vi "tag bus to profibus.vi"(10 "slave configuration":T2, 11 "data table in in":T1) -> (1 "Data":u8[](array[numeric]), 2 "slave index":i8, 3 "data table out":T1)   [LabVIEW 2013, in "Profibus Module runtime.lvclass"]
uses:
  Profibus Module runtime.lvclass
  profibus slave configuration.ctl
  profibus mapping configuration.ctl
  <vilib>/NI/Tag Bus/tag/Data Type.ctl
  <vilib>/NI/Tag Bus/table/data table.ctl
  <vilib>/NI/Tag Bus/table/data polymorphs/read one/read Double.vi
  <vilib>/NI/Tag Bus/table/data polymorphs/read one/read Single.vi
  <vilib>/NI/Tag Bus/table/data polymorphs/read one/read U32.vi
  <vilib>/NI/Tag Bus/table/data polymorphs/read one/read U16.vi
  <vilib>/NI/Tag Bus/table/data polymorphs/read one/read I16.vi
  <vilib>/NI/Tag Bus/table/data polymorphs/read one/read Array of U8.vi
  <vilib>/NI/Tag Bus/table/data polymorphs/read one/read Array of U32.vi
  <vilib>/NI/Tag Bus/table/data polymorphs/read one/read Array of U16.vi
  <vilib>/NI/Tag Bus/table/data polymorphs/read one/read U8.vi
  <vilib>/NI/Tag Bus/table/data polymorphs/read one/read I8.vi
  <vilib>/NI/Tag Bus/table/data polymorphs/read one/read Boolean.vi
  <vilib>/NI/Tag Bus/table/data table.lvlib
  <vilib>/NI/Tag Bus/tag/tag descriptor.lvclass
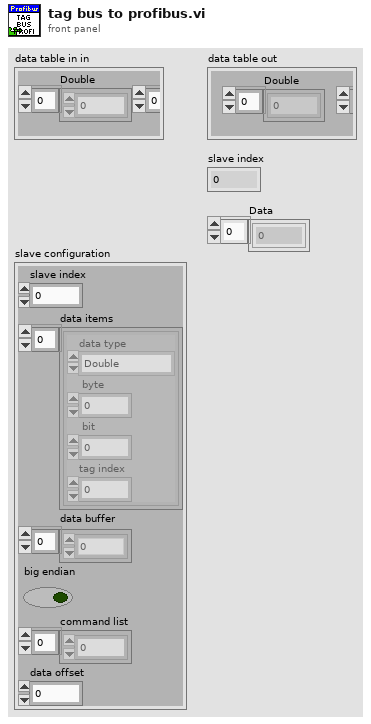
[diagram p1: front panel]
types:
  T1 = typedef "tag bus.lvlib/data table.lvlib/data table.ctl" = cluster{"Double":dbl[], "Single":sgl[], "I64":i64[], "I32":i32[], "I16":i16[], "I8":i8[], "U64":u64[], "U32":u32[], "U16":u16[], "U8":u8[], "Boolean":bool[], "String":string[], "Array of Double":cluster{"DBL Array":dbl[]}[], "Array of Single":cluster{"SGL Array":sgl[]}[], "Array of I64":cluster{"I64 Array":i64[]}[], "Array of I32":cluster{"I32 Array":i32[]}[], "Array of I16":cluster{"I16 Array":i16[]}[], "Array of I8":cluster{"I8 Array":i8[]}[], "Array of U64":cluster{"U64 Array":u64[]}[], "Array of U32":cluster{"U32 Array":u32[]}[], "Array of U16":cluster{"U16 Array":u16[]}[], "Array of U8":cluster{"U8 Array":u8[]}[], "Array of Boolean":cluster{"Boolean Array":bool[]}[], "Array of String":cluster{"String Array":string[]}[]}
  T2 = typedef "Profibus Module runtime.lvclass/profibus slave configuration.ctl" = cluster{"slave index":i8, "data items":T3[], "data buffer":u8[], "big endian":bool, "command list":u32[], "data offset":u8}
  T3 = typedef "Profibus Module runtime.lvclass/profibus mapping configuration.ctl" = cluster{"data type":T4, " byte":i32, " bit":i32, "tag index":i32}
  T4 = typedef "tag bus.lvlib/tag descriptor.lvclass/Data Type.ctl" = enum16{"Double", "Single", "I64", "I32", "I16", "I8", "U64", "U32", "U16", "U8", "Boolean", "String", "Array of Double", "Array of Single", "Array of I64", "Array of I32", "Array of I16", "Array of I8", "Array of U64", "Array of U32", "Array of U16", "Array of U8", "Array of Boolean", "Array of String"}
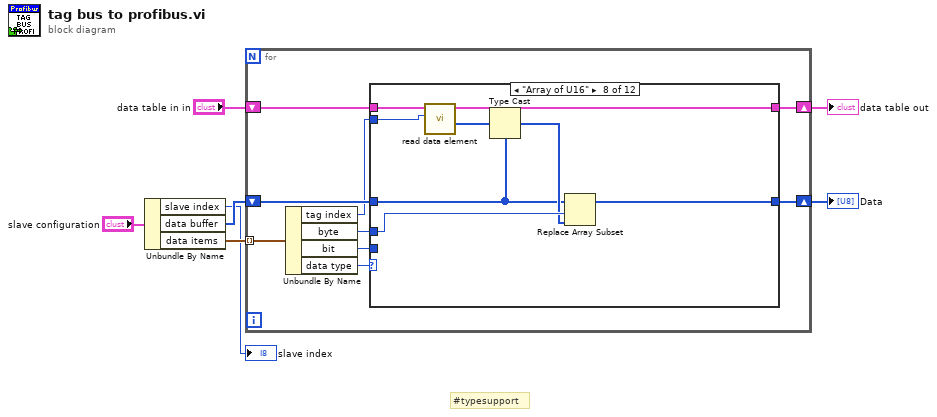
[diagram p0: block diagram]
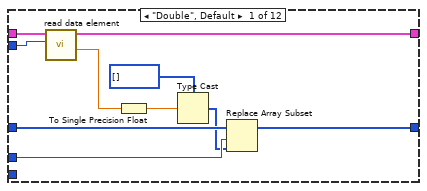
[diagram p2: hidden frame]
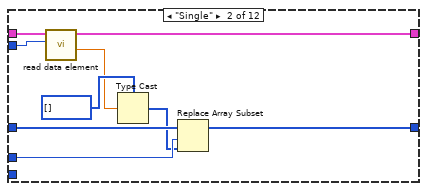
[diagram p3: hidden frame]
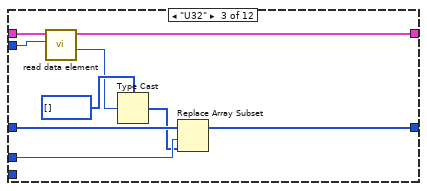
[diagram p4: hidden frame]
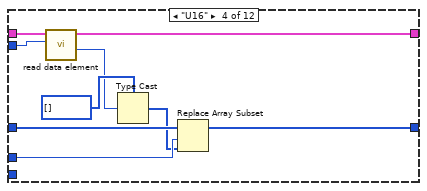
[diagram p5: hidden frame]
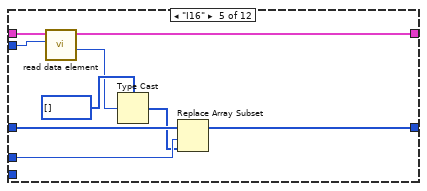
[diagram p6: hidden frame]
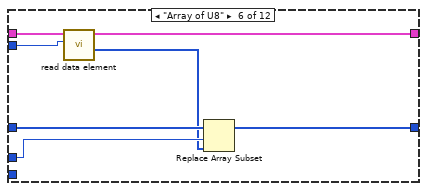
[diagram p7: hidden frame]
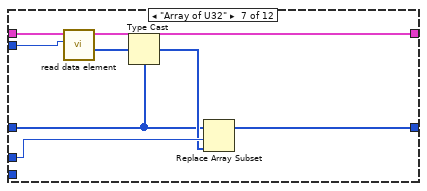
[diagram p8: hidden frame]
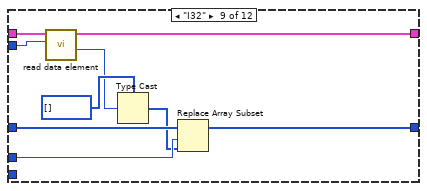
[diagram p9: hidden frame]
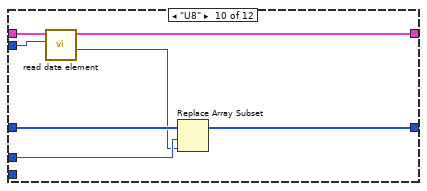
[diagram p10: hidden frame]
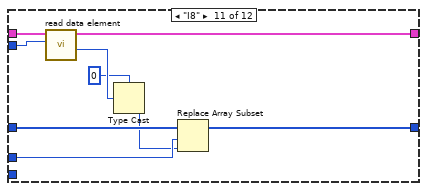
[diagram p11: hidden frame]
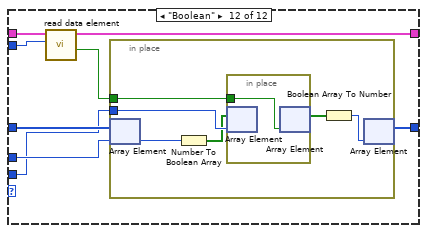
[diagram p12: hidden frame]
diagram:
  # "#typesupport"
  n1 = Unbundle By Name("slave configuration") -> ("slave index"=→"slave index":i8, "data buffer"=w6:u8[], "data items"=w4:T3[])
  n2 = for {
    tunnel: w4 -> [w16] mode=indexing
    shift-right: [w14] -> w5
    shift-left: w6 -> [w15]
    shift-right: [w9] -> w2
    shift-left: "data table in in" -> [w10]
    n3 = Unbundle By Name(w16) -> ("tag index"=w8:i32, "byte"=w13:i32, "bit"=w11:i32, "data type"=w12:T4)
    n4 = case shown="\"Array of U16\"" w12 {
      tunnel: w8 -> [w18 w28 w37 w46 w55 w68 w76 w84 w87 w96 w105 w111]
      tunnel: w15 -> [w24 w34 w43 w52 w61 w66 w70 w78 w93 w101 w110 w118]
      tunnel: w13 -> [w22 w32 w41 w50 w59 w64 w73 w81 w91 w99 w108 w117]
      tunnel: [w23 w33 w42 w51 w60 w65 w74 w82 w92 w100 w109 w116] -> w14
      tunnel: w11 -> [_ _ _ _ _ _ _ _ _ _ _ w115]
      tunnel: w10 -> [w20 w30 w39 w48 w57 w69 w77 w85 w89 w98 w107 w112]
      tunnel: [w19 w29 w38 w47 w56 w67 w75 w83 w88 w97 w106 w113] -> w9
      frame "Double", Default {
        n5 = call-poly <vilib>:"read data element.vi"("index"=w18, "data table in"=w20) -> ("value"=w17:dbl, "data table out"=w19:T1)  [unwired: 8 in]
        n6 = To Single Precision Float(number=w17) -> (single precision float=w25:sgl)
        n7 = Type Cast(type=u8[] [] ("Array 2"), x=w25) -> (*(type *) &x=w21:u8[])
        n8 = Replace Array Subset(array=w24, new element=w21, index=w22) -> (w23:u8[])
      }
      frame "Single" {
        n9 = call-poly <vilib>:"read data element.vi"("index"=w28, "data table in"=w30) -> ("value"=w27:sgl, "data table out"=w29:T1)  [unwired: 8 in]
        n10 = Type Cast(type=u8[] [] ("Array 2"), x=w27) -> (*(type *) &x=w31:u8[])
        n11 = Replace Array Subset(array=w34, new element=w31, index=w32) -> (w33:u8[])
      }
      frame "U32" {
        n12 = call-poly <vilib>:"read data element.vi"("index"=w37, "data table in"=w39) -> ("value"=w36:u32, "data table out"=w38:T1)  [unwired: 8 in]
        n13 = Type Cast(type=u8[] [] ("Array 2"), x=w36) -> (*(type *) &x=w40:u8[])
        n14 = Replace Array Subset(array=w43, new element=w40, index=w41) -> (w42:u8[])
      }
      frame "U16" {
        n15 = call-poly <vilib>:"read data element.vi"("index"=w46, "data table in"=w48) -> ("value"=w45:u16, "data table out"=w47:T1)  [unwired: 8 in]
        n16 = Type Cast(type=u8[] [] ("Array 2"), x=w45) -> (*(type *) &x=w49:u8[])
        n17 = Replace Array Subset(array=w52, new element=w49, index=w50) -> (w51:u8[])
      }
      frame "I16" {
        n18 = call-poly <vilib>:"read data element.vi"("index"=w55, "data table in"=w57) -> ("value"=w54:i16, "data table out"=w56:T1)  [unwired: 8 in]
        n19 = Type Cast(type=u8[] [] ("Array 2"), x=w54) -> (*(type *) &x=w58:u8[])
        n20 = Replace Array Subset(array=w61, new element=w58, index=w59) -> (w60:u8[])
      }
      frame "Array of U8" {
        n21 = call-poly <vilib>:"read data element.vi"("index"=w68, "data table in"=w69) -> ("value"=w63:u8[], "data table out"=w67:T1)  [unwired: 8 in]
        n22 = Replace Array Subset(array=w66, new element=w63, index=w64) -> (w65:u8[])
      }
      frame "Array of U32" {
        n23 = call-poly <vilib>:"read data element.vi"("index"=w76, "data table in"=w77) -> ("value"=w72:u32[], "data table out"=w75:T1)  [unwired: 8 in]
        n24 = Type Cast(type=w70, x=w72) -> (*(type *) &x=w71:u8[])
        n25 = Replace Array Subset(array=w70, new element=w71, index=w73) -> (w74:u8[])
      }
      frame "Array of U16" {
        n26 = call-poly <vilib>:"read data element.vi"("index"=w84, "data table in"=w85) -> ("value"=w80:u16[], "data table out"=w83:T1)  [unwired: 8 in]
        n27 = Type Cast(type=w78, x=w80) -> (*(type *) &x=w79:u8[])
        n28 = Replace Array Subset(array=w78, new element=w79, index=w81) -> (w82:u8[])
      }
      frame "I32" {
        n29 = call-poly <vilib>:"read data element.vi"("index"=w87, "data table in"=w89) -> ("value"=w86:u32, "data table out"=w88:T1)  [unwired: 8 in]
        n30 = Type Cast(type=u8[] [] ("Array 2"), x=w86) -> (*(type *) &x=w90:u8[])
        n31 = Replace Array Subset(array=w93, new element=w90, index=w91) -> (w92:u8[])
      }
      frame "U8" {
        n32 = call-poly <vilib>:"read data element.vi"("index"=w96, "data table in"=w98) -> ("value"=w95:u8, "data table out"=w97:T1)  [unwired: 8 in]
        n33 = Replace Array Subset(array=w101, new element=w95, index=w99) -> (w100:u8[])
      }
      frame "I8" {
        n34 = call-poly <vilib>:"read data element.vi"("index"=w105, "data table in"=w107) -> ("value"=w103:i8, "data table out"=w106:T1)  [unwired: 8 in]
        n35 = Type Cast(type=i8 0, x=w103) -> (*(type *) &x=w104:i8)
        n36 = Replace Array Subset(array=w110, new element=w104, index=w108) -> (w109:u8[])
      }
      frame "Boolean" {
        n37 = call-poly <vilib>:"read data element.vi"("index"=w111, "data table in"=w112) -> ("value"=w114:bool, "data table out"=w113:T1)  [unwired: 8 in]
        n38 = in-place {
          in-place-border: w115 -> [w123]
          in-place-border: w114 -> [w122]
          n39 = in-place-array #1(w118, w117) -> (w124:u8)
          n40 = Number To Boolean Array(number=w124) -> (Boolean array=w119:bool[])
          n41 = in-place {
            in-place-border: w122 -> [w125]
            n42 = in-place-array #2(w119, w123) -> ()  [unwired: 1 out]
            n43 = in-place-array #2(w125) -> (w120:bool[])  [unwired: 1 out]
          }
          n44 = Boolean Array To Number(Boolean array=w120) -> (number=w121:u8)
          n45 = in-place-array #1(w121) -> (w116:u8[])  [unwired: 1 out]
        }
      }
    }
  }
  "Data" <- w5
  "data table out" <- w2
